vi "Interpret Driver Actions.vi"(10 "loop time manipulator (ms)":u32=10, 11 "loop time driver (ms)":u32=10) -> ()   [LabVIEW 2017]
uses:
  <vilib>/Rock Robotics/WPI/DriverStation/WPI_DriverStationRobotMode2.ctl
  <vilib>/Rock Robotics/WPI/Solenoid/WPI_SolenoidValue.ctl
  <vilib>/Rock Robotics/WPI/Utilities/WPI_GetSetVariantRefNum.vi
  Globals/Robot Global Data.vi
  Globals/Driver Controller Inputs.vi
  Globals/Manipulator Controller Inputs.vi
  <vilib>/express/express arith-compare/Formula/XNode/ExpressFormulaBlockNode.xnode
panel:
  in  "Left Rumble":sgl=0.4
  in  "Right Rumble":sgl=0.4
  in  "Distance from Setpoint Override":dbl=12.0
  in  "Turn on auto cube up":bool
  in  "Driver Slowdown X":dbl=0.65
  in  "Driver Slowdown Y":dbl=0.8
  in  "Outake Speed":dbl=-3.0 format="%#_13g"
  in  "Intake Speed":dbl=1.0
  in  "Drive Y Scalar":dbl=3.0
  in  "Drive X Scalar":dbl=3.0
  in  "Drive X Multilpier":dbl=0.9
  in  "Drive Y Multilpier":dbl=0.9
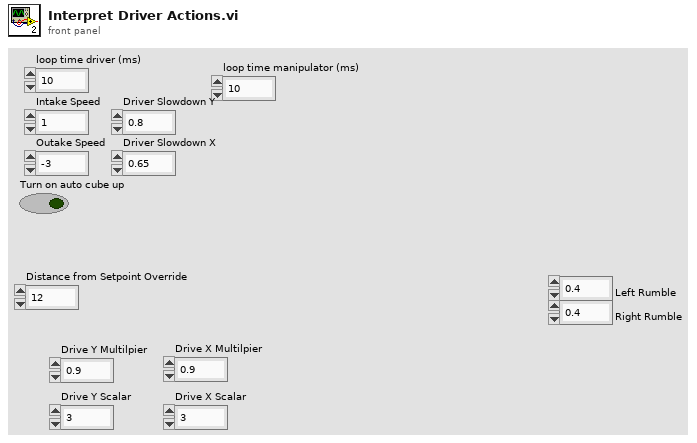
[diagram p1: front panel]
types:
  T1 = typedef "WPI_JoystickDevRef.ctl" = cluster{"Device":T2}
  T2 = typedef "WPI_JoystickDeviceEnum.ctl" = enum16{"USB 0", "USB 1", "USB 2", "USB 3", "USB 4", "USB 5"}
  T3 = typedef "WPI_DriverStationRobotMode2.ctl" = enum16{"Autonomous Disabled", "Autonomous Enabled", "Teleop Disabled", "Teleop Enabled", "Disconnected", "Finish", "Test Disabled", "Test Enabled", "Emergency Stopped"}
  T4 = typedef "WPI_SolenoidValue.ctl" = enum16{"Off", "On", "Forward", "Reverse"}
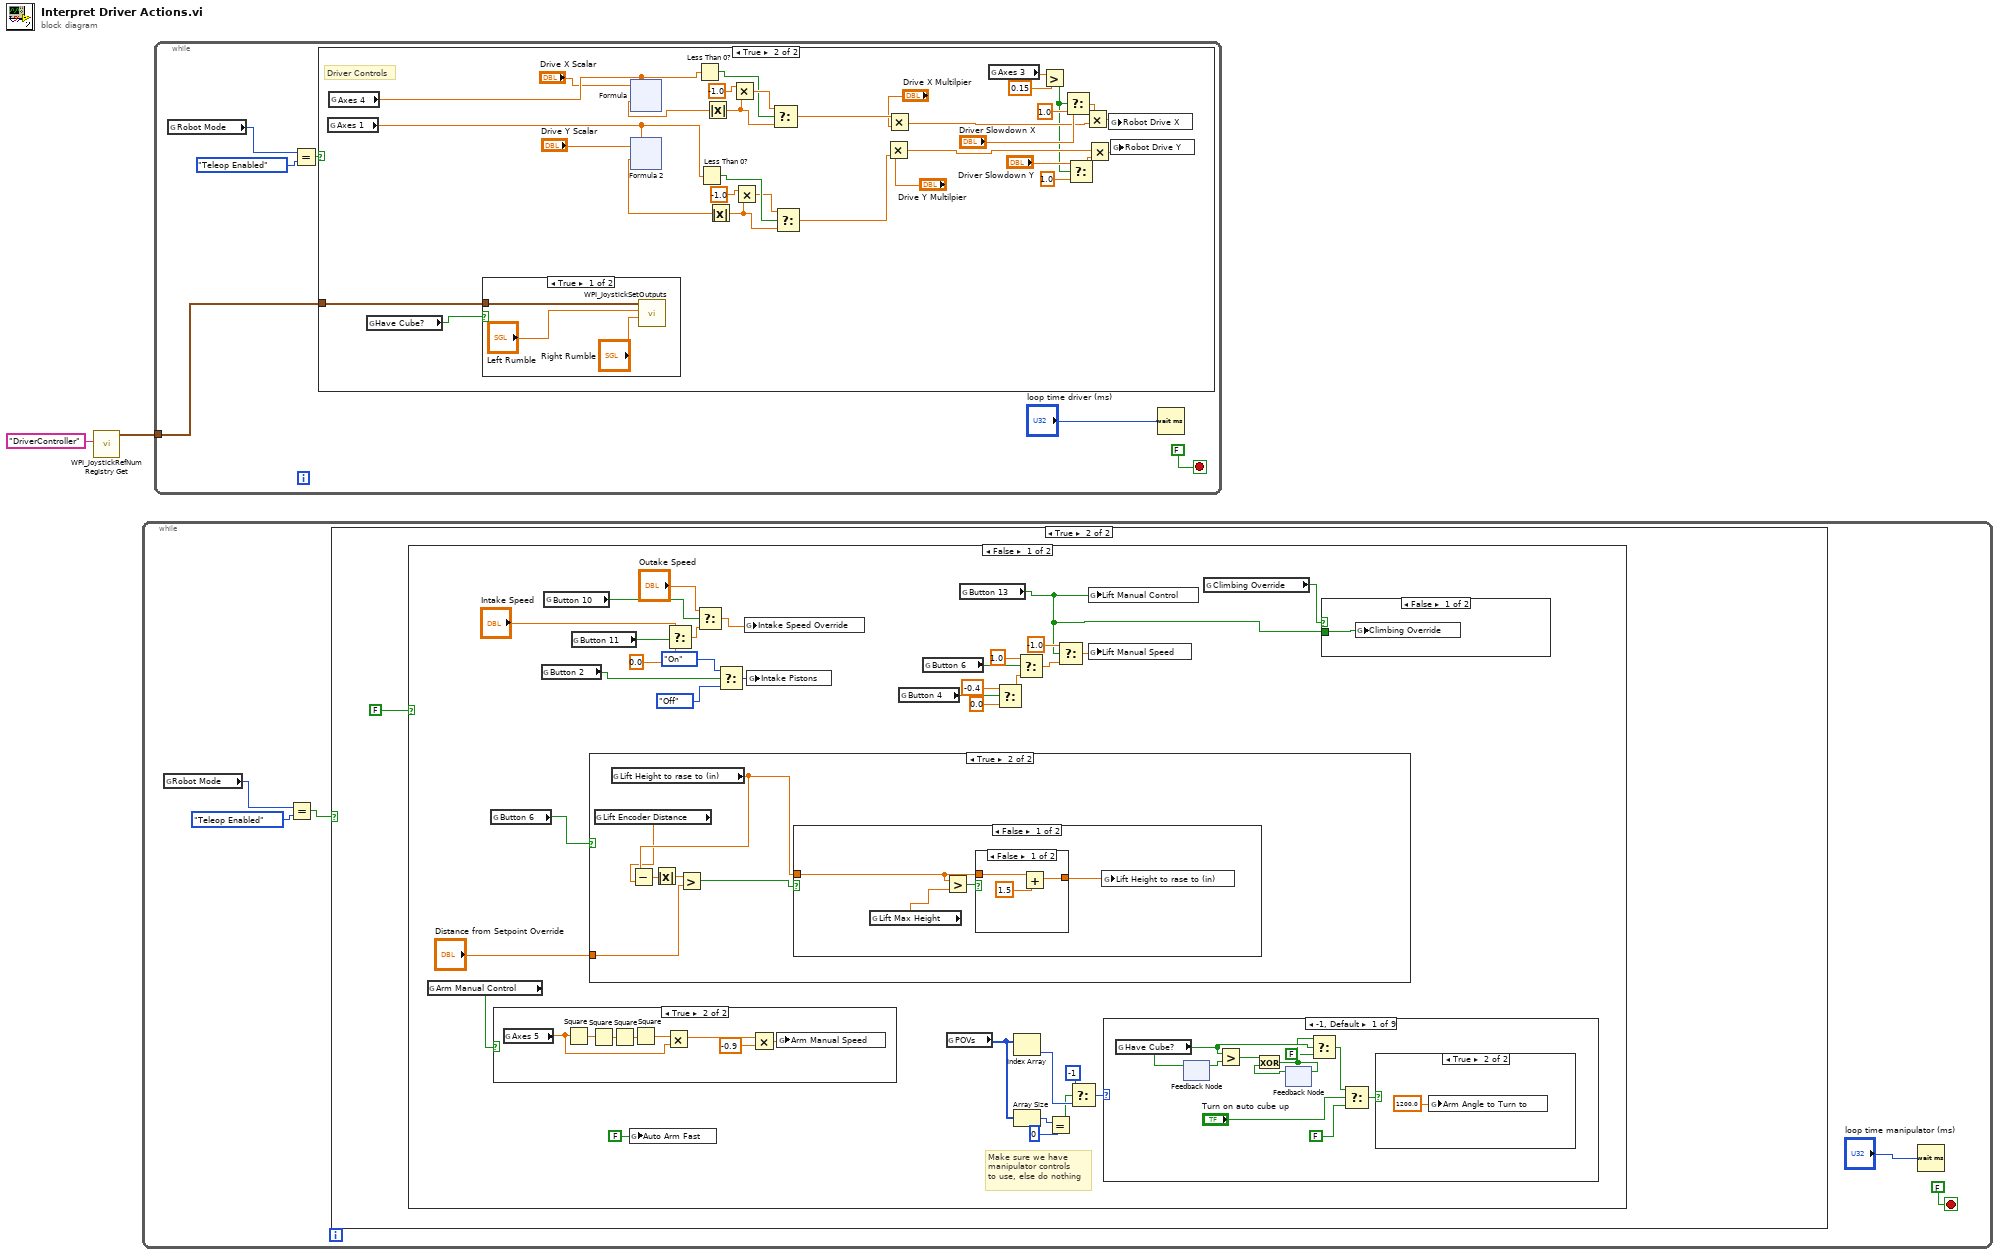
[diagram p0: block diagram]
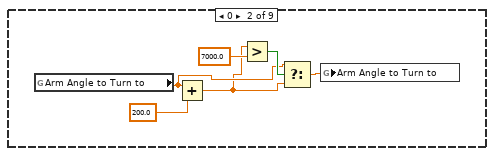
[diagram p4: hidden frame]
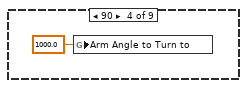
[diagram p6: hidden frame]
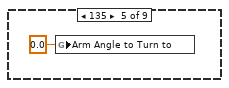
[diagram p7: hidden frame]
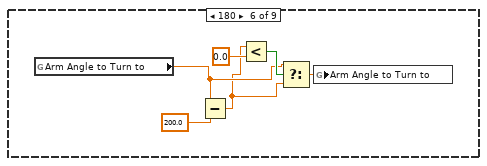
[diagram p8: hidden frame]
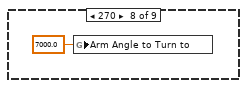
[diagram p10: hidden frame]
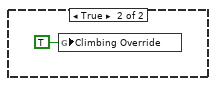
[diagram p12: hidden frame]
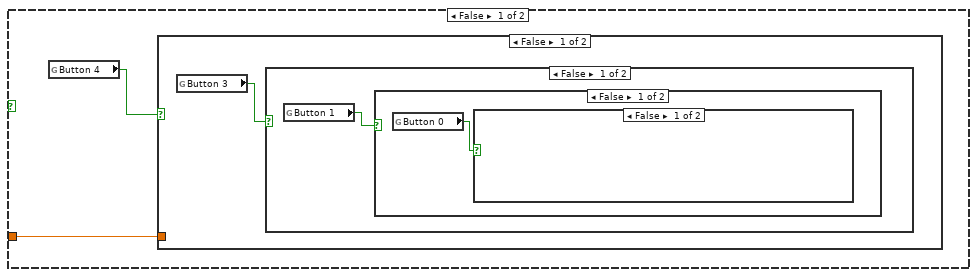
[diagram p14: hidden frame]
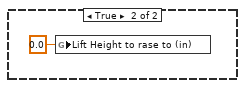
[diagram p15: hidden frame]
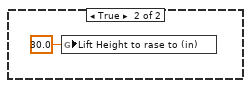
[diagram p16: hidden frame]
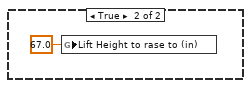
[diagram p17: hidden frame]
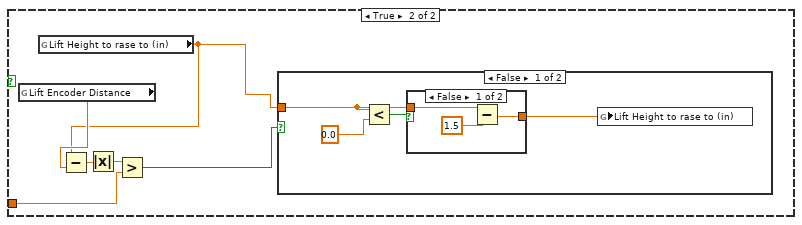
[diagram p18: hidden frame]
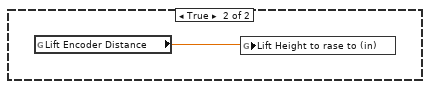
[diagram p20: hidden frame]
diagram:
  n1 = call <vilib>:"WPI_JoystickRefNum Registry Get.vi"("refnum name"="DriverController") -> ("JoystickDevRef"=w1:T1)  [unwired: 9 in, 1 out]
  n2 = while {
    stop <- FALSE stop-if-true
    n3 = global read "Robot Global Data.vi" "Robot Mode"() -> (w4:T3)
    n4 = Equal?(x=w4, y=WPI_DriverStationRobotMode2."Teleop Enabled" ("Robot Mode")) -> (x = y?=w3:bool)
    n5 = case shown="True" w3 {
      frame False {
      }
      frame True {
        n6 = case shown="False" FALSE {
          frame False {
            # "Make sure we have\nmanipulator controls\nto use, else do nothing"
            n7 = global read "Robot Global Data.vi" "Arm Manual Control"() -> (w27:bool)
            n8 = global read "Manipulator Controller Inputs.vi" "Button 6"() -> (w30:bool)
            n9 = case shown="True" w27 {
              frame False {
              }
              frame True {
                n10 = global read "Manipulator Controller Inputs.vi" "Axes 5"() -> (w73:dbl)
                n11 = Square(x=w73) -> (x^2=w77:dbl)
                n12 = Square(x=w77) -> (x^2=w76:dbl)
                n13 = Square(x=w76) -> (x^2=w75:dbl)
                n14 = Square(x=w75) -> (x^2=w74:dbl)
                n15 = Multiply(x=w74, y=w73) -> (x*y=w72:dbl)
                n16 = Multiply(x=w72, y=-0.9) -> (x*y=w71:dbl)
                n17 = global write "Robot Global Data.vi" "Arm Manual Speed"(w71) -> ()
              }
            }
            n18 = global read "Manipulator Controller Inputs.vi" "Button 2"() -> (w35:bool)
            n19 = global read "Manipulator Controller Inputs.vi" "Button 10"() -> (w41:bool)
            n20 = global read "Manipulator Controller Inputs.vi" "Button 11"() -> (w31:bool)
            n21 = case shown="True" w30 {
              tunnel: "Distance from Setpoint Override" -> [w78 w101]
              frame False {
                n22 = global read "Manipulator Controller Inputs.vi" "Button 4"() -> (w79:bool)
                n23 = case shown="False" w79 {
                  tunnel: w78 -> [_ w86]
                  frame False {
                    n24 = global read "Manipulator Controller Inputs.vi" "Button 3"() -> (w80:bool)
                    n25 = case shown="False" w80 {
                      frame False {
                        n26 = global read "Manipulator Controller Inputs.vi" "Button 1"() -> (w81:bool)
                        n27 = case shown="False" w81 {
                          frame False {
                            n28 = global read "Manipulator Controller Inputs.vi" "Button 0"() -> (w82:bool)
                            n29 = case shown="False" w82 {
                              frame False {
                              }
                              frame True {
                                n30 = global write "Robot Global Data.vi" "Lift Height to rase to (in)"(0.0 ("Lift Height to rase to (in)")) -> ()
                              }
                            }
                          }
                          frame True {
                            n31 = global write "Robot Global Data.vi" "Lift Height to rase to (in)"(30.0 ("Lift Height to rase to (in)")) -> ()
                          }
                        }
                      }
                      frame True {
                        n32 = global write "Robot Global Data.vi" "Lift Height to rase to (in)"(67.0 ("Lift Height to rase to (in)")) -> ()
                      }
                    }
                  }
                  frame True {
                    n33 = global read "Robot Global Data.vi" "Lift Encoder Distance"() -> (w91:dbl)
                    n34 = global read "Robot Global Data.vi" "Lift Height to rase to (in)"() -> (w88:dbl)
                    n35 = Subtract(x=w88, y=w91) -> (x-y=w90:dbl)
                    n36 = Absolute Value(x=w90) -> (abs(x)=w89:dbl)
                    n37 = Greater?(x=w89, y=w86) -> (0:w87:bool)
                    n38 = case shown="False" w87 {
                      tunnel: w88 -> [w92 _]
                      frame False {
                        n39 = Less?(x=w92, y=0.0) -> (x < y?=w94:bool)
                        n40 = case shown="False" w94 {
                          tunnel: w92 -> [w98 w99]
                          tunnel: [w96 w99] -> w95
                          frame False {
                            n41 = Subtract(x=w98, y=1.5) -> (x-y=w96:dbl)
                          }
                          frame True {
                          }
                        }
                        n42 = global write "Robot Global Data.vi" "Lift Height to rase to (in)"(w95) -> ()
                      }
                      frame True {
                        n43 = global read "Robot Global Data.vi" "Lift Encoder Distance"() -> (w100:dbl)
                        n44 = global write "Robot Global Data.vi" "Lift Height to rase to (in)"(w100) -> ()
                      }
                    }
                  }
                }
              }
              frame True {
                n45 = global read "Robot Global Data.vi" "Lift Encoder Distance"() -> (w105:dbl)
                n46 = global read "Robot Global Data.vi" "Lift Height to rase to (in)"() -> (w106:dbl)
                n47 = Subtract(x=w106, y=w105) -> (x-y=w104:dbl)
                n48 = Absolute Value(x=w104) -> (abs(x)=w103:dbl)
                n49 = Greater?(x=w103, y=w101) -> (0:w102:bool)
                n50 = case shown="False" w102 {
                  tunnel: w106 -> [w108 _]
                  frame False {
                    n51 = global read "Robot Global Data.vi" "Lift Max Height"() -> (w107:dbl)
                    n52 = Greater?(x=w108, y=w107) -> (0:w109:bool)
                    n53 = case shown="False" w109 {
                      tunnel: w108 -> [w113 w114]
                      tunnel: [w111 w114] -> w110
                      frame False {
                        n54 = Add(x=w113, y=1.5) -> (x+y=w111:dbl)
                      }
                      frame True {
                      }
                    }
                    n55 = global write "Robot Global Data.vi" "Lift Height to rase to (in)"(w110) -> ()
                  }
                  frame True {
                    n56 = global read "Robot Global Data.vi" "Lift Encoder Distance"() -> (w115:dbl)
                    n57 = global write "Robot Global Data.vi" "Lift Height to rase to (in)"(w115) -> ()
                  }
                }
              }
            }
            n58 = global write "Robot Global Data.vi" "Auto Arm Fast"(FALSE ("Auto Arm Fast")) -> ()
            n59 = Select(t="Intake Speed", s=w31, f=0.0) -> (s? t:f=w34:dbl)
            n60 = Select(t="Outake Speed", s=w41, f=w34) -> (s? t:f=w40:dbl)
            n61 = Select(t=WPI_SolenoidValue."On" ("Intake Pistons"), s=w35, f=WPI_SolenoidValue."Off" ("Intake Pistons")) -> (s? t:f=w37:T4)
            n62 = global write "Robot Global Data.vi" "Intake Speed Override"(w40) -> ()
            n63 = global write "Robot Global Data.vi" "Intake Pistons"(w37) -> ()
            n64 = global read "Manipulator Controller Inputs.vi" "Button 4"() -> (w25:bool)
            n65 = global read "Manipulator Controller Inputs.vi" "Button 6"() -> (w26:bool)
            n66 = global read "Manipulator Controller Inputs.vi" "POVs"() -> (w17:i16[])
            n67 = global read "Manipulator Controller Inputs.vi" "Button 13"() -> (w18:bool)
            n68 = Select(t=-0.4, s=w25, f=0.0) -> (s? t:f=w24:dbl)
            n69 = Index Array(array=w17) -> (element=w15:i16)  [unwired: 1 in]
            n70 = Array Size(array=w17) -> (size(s)=w13:i32)
            n71 = Select(t=1.0, s=w26, f=w24) -> (s? t:f=w23:dbl)
            n72 = Equal?(x=w13, y=0) -> (x = y?=w11:bool)
            n73 = Select(t=-1.0, s=w18, f=w23) -> (s? t:f=w29:dbl)
            n74 = Select(t=i16 -1, s=w11, f=w15) -> (s? t:f=w16:i16)
            n75 = global write "Robot Global Data.vi" "Lift Manual Control"(w18) -> ()
            n76 = global write "Robot Global Data.vi" "Lift Manual Speed"(w29) -> ()
            n77 = case shown="-1, Default" w16 {
              frame -1, Default {
                n78 = global read "Robot Global Data.vi" "Have Cube?"() -> (w45:bool)
                n79 = feedback-in #1(w45) -> ()
                n80 = feedback #1() -> (w51:bool)  [unwired: 1 in]
                n81 = Greater?(x=w45, y=w51) -> (0:w50:bool)
                n82 = feedback #2() -> (w49:bool)  [unwired: 1 in]
                n83 = Exclusive Or(1:w49, 2:w50) -> (0:w44:bool)
                n84 = feedback-in #2(w44) -> ()
                n85 = Select(t=w44, s=w45, f=FALSE) -> (s? t:f=w42:bool)
                n86 = Select(t=w42, s="Turn on auto cube up", f=FALSE) -> (s? t:f=w48:bool)
                n87 = case shown="True" w48 {
                  frame False {
                  }
                  frame True {
                    n88 = global write "Robot Global Data.vi" "Arm Angle to Turn to"(1200.0 ("Arm Angle to Turn to")) -> ()
                  }
                }
              }
              frame 0 {
                n89 = global read "Robot Global Data.vi" "Arm Angle to Turn to"() -> (w54:dbl)
                n90 = Add(x=w54, y=200.0) -> (x+y=w53:dbl)
                n91 = Greater?(x=w53, y=7000.0) -> (0:w56:bool)
                n92 = Select(t=w54, s=w56, f=w53) -> (s? t:f=w55:dbl)
                n93 = global write "Robot Global Data.vi" "Arm Angle to Turn to"(w55) -> ()
              }
              frame 45 {
              }
              frame 90 {
                n94 = global write "Robot Global Data.vi" "Arm Angle to Turn to"(1000.0 ("Arm Angle to Turn to")) -> ()
              }
              frame 135 {
                n95 = global write "Robot Global Data.vi" "Arm Angle to Turn to"(0.0 ("Arm Angle to Turn to")) -> ()
              }
              frame 180 {
                n96 = global read "Robot Global Data.vi" "Arm Angle to Turn to"() -> (w62:dbl)
                n97 = Subtract(x=w62, y=200.0) -> (x-y=w61:dbl)
                n98 = Less?(x=w61, y=0.0) -> (x < y?=w64:bool)
                n99 = Select(t=w62, s=w64, f=w61) -> (s? t:f=w63:dbl)
                n100 = global write "Robot Global Data.vi" "Arm Angle to Turn to"(w63) -> ()
              }
              frame 225 {
              }
              frame 270 {
                n101 = global write "Robot Global Data.vi" "Arm Angle to Turn to"(7000.0 ("Arm Angle to Turn to")) -> ()
              }
              frame 315 {
              }
            }
            n102 = global read "Robot Global Data.vi" "Climbing Override"() -> (w19:bool)
            n103 = case shown="False" w19 {
              tunnel: w18 -> [w68 _]
              frame False {
                n104 = global write "Robot Global Data.vi" "Climbing Override"(w68) -> ()
              }
              frame True {
                n105 = global write "Robot Global Data.vi" "Climbing Override"(TRUE ("Climbing Override")) -> ()
              }
            }
          }
          frame True {
          }
        }
      }
    }
    n106 = Wait (ms)(milliseconds to wait="loop time manipulator (ms)") -> ()  [unwired: 1 out]
  }
  n107 = while {
    tunnel: w1 -> [w116]
    stop <- FALSE stop-if-true
    n108 = global read "Robot Global Data.vi" "Robot Mode"() -> (w117:T3)
    n109 = Equal?(x=w117, y=WPI_DriverStationRobotMode2."Teleop Enabled" ("Robot Mode")) -> (x = y?=w119:bool)
    n110 = case shown="True" w119 {
      tunnel: w116 -> [_ w122]
      frame False {
      }
      frame True {
        # "Driver Controls"
        n111 = global read "Driver Controller Inputs.vi" "Axes 1"() -> (w143:dbl)
        n112 = global read "Driver Controller Inputs.vi" "Axes 4"() -> (w153:dbl)
        n113 = global read "Robot Global Data.vi" "Have Cube?"() -> (w123:bool)
        n114 = case shown="True" w123 {
          tunnel: w122 -> [w157 w159]
          frame True {
            n115 = call <vilib>:"WPI_JoystickSetOutputs.vi"("Right Rumble"="Right Rumble", "Left Rumble"="Left Rumble", "JoystickDevRef"=w157) -> ()  [unwired: 7 in, 2 out]
          }
          frame False {
            w158 = sgl 0.0 ("Left Rumble")
            n116 = call <vilib>:"WPI_JoystickSetOutputs.vi"("Right Rumble"=w158, "Left Rumble"=w158, "JoystickDevRef"=w159) -> ()  [unwired: 7 in, 2 out]
          }
        }
        n117 = xnode ("Formula")("Scalar"="Drive X Scalar", "Original"=w153) -> ("Result"=w154:dbl)  [unwired: 1 in, 1 out]
        n118 = xnode ("Formula 2")("Scalar"="Drive Y Scalar", "Original"=w143) -> ("Result"=w142:dbl)  [unwired: 1 in, 1 out]
        n119 = Less Than 0?(x=w153) -> (x < 0?=w150:bool)
        n120 = Less Than 0?(x=w143) -> (x < 0?=w146:bool)
        n121 = Absolute Value(x=w154) -> (abs(x)=w149:dbl)
        n122 = Absolute Value(x=w142) -> (abs(x)=w147:dbl)
        n123 = Multiply(x=-1.0, y=w149) -> (x*y=w151:dbl)
        n124 = Multiply(x=-1.0, y=w147) -> (x*y=w145:dbl)
        n125 = Select(t=w151, s=w150, f=w149) -> (s? t:f=w148:dbl)
        n126 = Select(t=w145, s=w146, f=w147) -> (s? t:f=w141:dbl)
        n127 = Multiply(x="Drive Y Multilpier", y=w141) -> (x*y=w128:dbl)
        n128 = Multiply(x=w148, y="Drive X Multilpier") -> (x*y=w126:dbl)
        n129 = global read "Driver Controller Inputs.vi" "Axes 3"() -> (w136:dbl)
        n130 = Greater?(x=w136, y=0.15) -> (0:w124:bool)
        n131 = Select(t="Driver Slowdown X", s=w124, f=1.0) -> (s? t:f=w127:dbl)
        n132 = Select(t="Driver Slowdown Y", s=w124, f=1.0) -> (s? t:f=w129:dbl)
        n133 = Multiply(x=w127, y=w126) -> (x*y=w125:dbl)
        n134 = Multiply(x=w128, y=w129) -> (x*y=w130:dbl)
        n135 = global write "Robot Global Data.vi" "Robot Drive X"(w125) -> ()
        n136 = global write "Robot Global Data.vi" "Robot Drive Y"(w130) -> ()
      }
    }
    n137 = Wait (ms)(milliseconds to wait="loop time driver (ms)") -> ()  [unwired: 1 out]
  }
